vi "genStimRandStreamStimulation.vi"(8 "error in (no error)":errorcluster, 11 "Stimulus in":refnum<class "Stimulus.lvclass">) -> (0 "error out":errorcluster, 3 "Stimulus out":refnum<class "Stimulus.lvclass">)   [LabVIEW 2014, in "Stimulus.lvclass"]
uses:
  Stimulus.lvclass
  Stimulus.lvclass/Stimulus.ctl
  <vilib>/Analysis/1siggen.llb/Riffle Array (I32).vi
  <vilib>/Analysis/NI_AALBase.lvlib
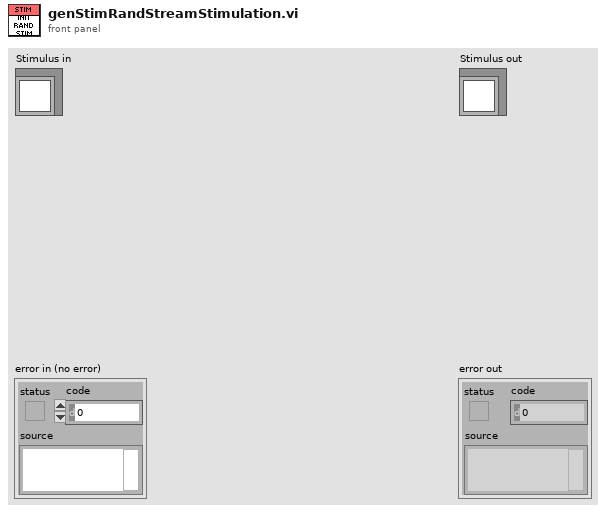
[diagram p1: front panel]
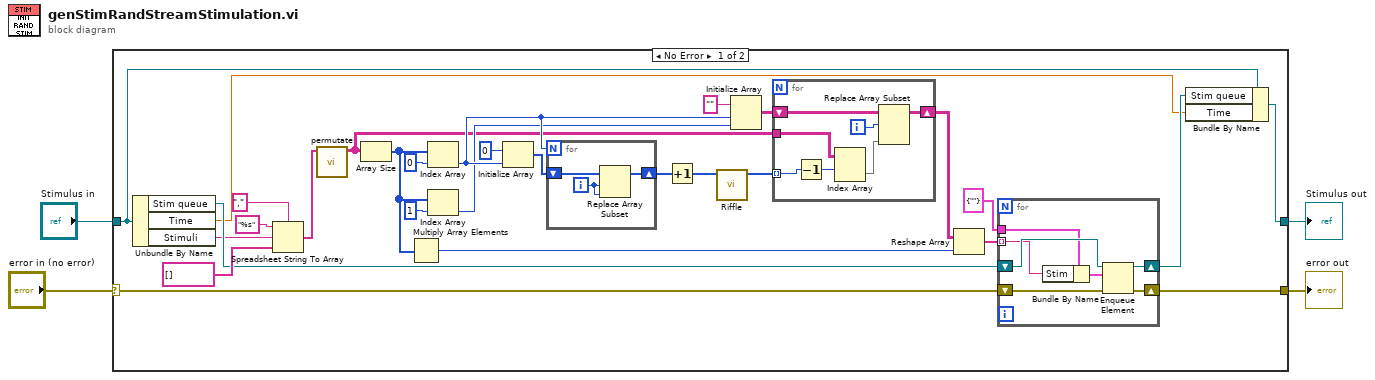
[diagram p0: block diagram]
diagram:
  n1 = case shown="No Error" "error in (no error)" {
    selector: "error in (no error)" -> [w33 w52]
    tunnel: [w32 w52] -> w3
    tunnel: [w6 w51] -> w1
    tunnel: "Stimulus in" -> [w7 w51]
    frame No Error {
      n2 = Unbundle By Name(w7) -> ("Stim queue"=w10:refnum<queue>, "Time"=w8:dbl, "Stimuli"=w5:string)
      n3 = Spreadsheet String To Array(delimiter (Tab)=",", format string="%s", spreadsheet string=w5, array type (2D Dbl)=string[] []) -> (array=w28:string[])
      n4 = call "permutate.vi"("Input"=w28) -> ("Permutations"=w16:string[][])  [unwired: 10 in]
      n5 = Array Size(array=w16) -> (size(s)=w15:i32[])
      n6 = Multiply Array Elements(1:w15) -> (0:w14:i32)
      n7 = Index Array(array=w15, index=0) -> (element=w21:i32)
      n8 = Index Array(array=w15, index=1) -> (element=w19:i32)
      n9 = Initialize Array(0, w21) -> (w25:i32[])
      n10 = for {
        N: w21 -> [_]
        shift-right: [w48] -> w24
        shift-left: w25 -> [w50]
        i -> [w49]
        n11 = Replace Array Subset(array=w50, new element=w49, index=w49) -> (w48:i32[])
      }
      n12 = Increment(x=w24) -> (x+1=w23:i32[])
      n13 = call-poly <vilib>:"Riffle.vi"("X"=w23) -> ("Riffled {X}"=w22:i32[])  [unwired: 8 in, 2 out]
      n14 = Initialize Array("", w21, w19) -> (w18:string[][])
      n15 = for {
        tunnel: w22 -> [w44] mode=indexing
        tunnel: w16 -> [w47]
        shift-right: [w42] -> w13
        shift-left: w18 -> [w45]
        i -> [w46]
        n16 = Decrement(x=w44) -> (x-1=w43:i32)
        n17 = Index Array(array=w47, index (row)=w43) -> (element=w41:string[])  [unwired: 1 in]
        n18 = Replace Array Subset(array=w45, new element=w41, index (row)=w46) -> (w42:string[][])  [unwired: 1 in]
      }
      n19 = Reshape Array(w13, w14) -> (w11:string[])
      n20 = for {
        shift-right: [w39] -> w32
        shift-left: w33 -> [w40]
        shift-right: [w37] -> w9
        shift-left: w10 -> [w38]
        tunnel: cluster{"Stim":string} {"Stim"=""} ("Stim element") -> [w36]
        tunnel: w11 -> [w35] mode=indexing
        n21 = Bundle By Name(cluster=w36, "Stim"=w35) -> (w34:cluster{"Stim":string})
        n22 = Enqueue Element(queue=w38, element=w34, error in (no error)=w40) -> (queue out=w37:refnum<queue>, error out=w39:errorcluster)  [unwired: 1 in, 1 out]
      }
      n23 = Bundle By Name(cluster=w7, "Stim queue"=w9, "Time"=w8) -> (w6:refnum<class "Stimulus.lvclass">)
    }
    frame Error {
    }
  }
  "error out" <- w3
  "Stimulus out" <- w1
